vi "xiCMNG - Manager.vi"(6 "xiCam":refnum<k24>, 7 "States":T1, 8 "error in (no error)":errorcluster, 10 "SubPnl":refnum<vi>, 11 "xiControlPath":path) -> (0 "error out":errorcluster, 3 "StatusOut":T2)   [LabVIEW 2013]
doc: "xiControl Manger. Action Engine for xiControl panel."
uses:
  xiCMNG - States.ctl
  xiCMNG - Attributes.ctl
  C:/Projects/Cameras3.x/xiLib/xiLIB_64bit/xiLIB/xiCamLib/API/x64/xiApi.NETX64.dll
  xiLIB_64bit/xiLIB/xiCamLib/API/x64/xiApi.NETX64.dll
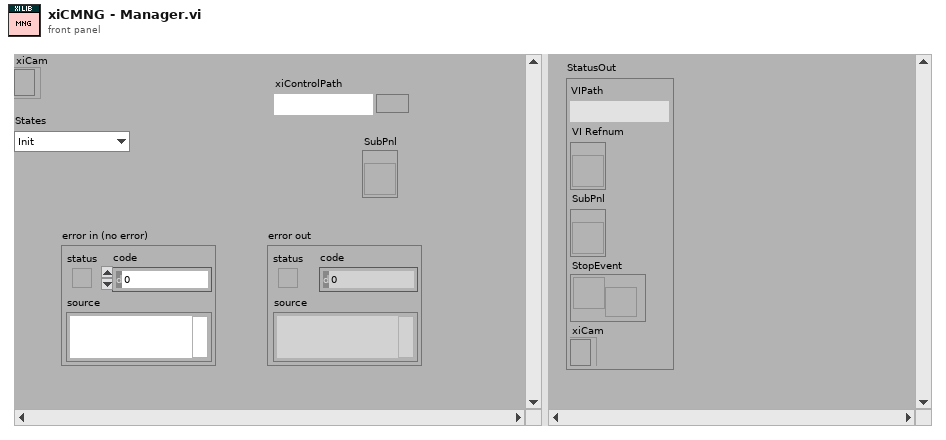
[diagram p1: front panel]
types:
  T1 = typedef "xiCMNG - States.ctl" = enum16{"Init", "Open", "Close", "Status"}
  T2 = typedef "xiCMNG - Attributes.ctl" = cluster{"VIPath":path, "VI Refnum":refnum<vi>, "SubPnl":refnum<vi>, "StopEvent":refnum<user-event>, "xiCam":refnum<k24>}
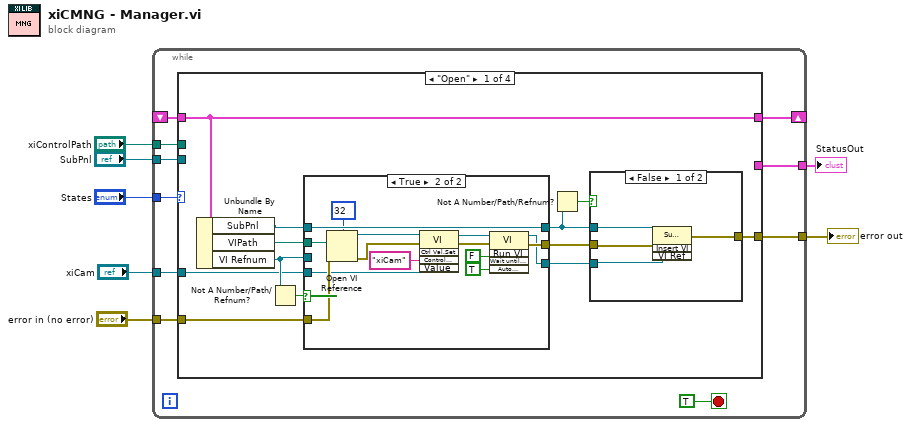
[diagram p0: block diagram]
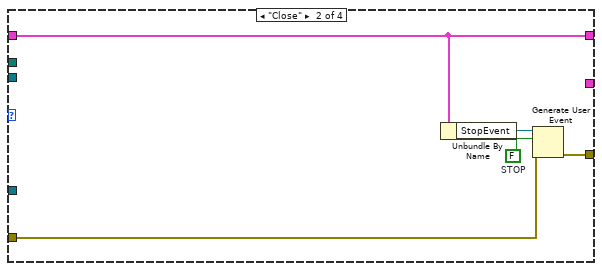
[diagram p4: hidden frame]
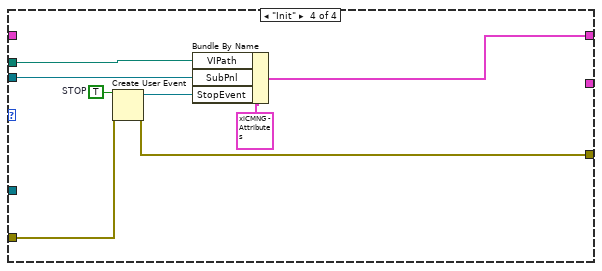
[diagram p6: hidden frame]
diagram:
  n1 = while {
    shift-right: [w16] -> _
    shift-left: _ -> [w10]
    tunnel: "States" -> [w15]
    tunnel: "error in (no error)" -> [w14]
    tunnel: [w13] -> w5
    tunnel: "SubPnl" -> [w12]
    tunnel: "xiControlPath" -> [w11]
    tunnel: [w9] -> w2
    tunnel: "xiCam" -> [w8]
    stop <- TRUE stop-if-true
    n2 = case shown="\"Open\"" w15 {
      tunnel: [w29 w56 w58 w63] -> w16
      tunnel: w14 -> [w26 w54 w57 w65]
      tunnel: [w19 w53 w57 w64] -> w13
      tunnel: w12 -> [_ _ _ w60]
      tunnel: w11 -> [_ _ _ w59]
      tunnel: w10 -> [w29 w56 w58 _]
      tunnel: [_ _ w58 _] -> w9
      tunnel: w8 -> [w18 _ _ _]
      frame "Open" {
        n3 = Unbundle By Name(w29) -> ("SubPnl"=w25:refnum<vi>, "VIPath"=w27:path, "VI Refnum"=w24:refnum<vi>)
        n4 = Not A Number/Path/Refnum?(number/path/refnum=w24) -> (NaN/Path/Refnum?=w28:bool)
        n5 = case shown="True" w28 {
          tunnel: w27 -> [_ w51]
          tunnel: w26 -> [w35 w50]
          tunnel: w25 -> [w36 w49]
          tunnel: [w36 w49] -> w22
          tunnel: [w37 w39] -> w20
          tunnel: w24 -> [w37 _]
          tunnel: [w35 w40] -> w21
          tunnel: w18 -> [_ w44]
          frame False {
          }
          frame True {
            n6 = Open VI Reference(vi path=w51, options=32, error in (no error)=w50) -> (vi reference=w47:refnum<vi>, error out=w46:errorcluster)  [unwired: 3 in]
            n7 = invoke class="VI" method="Ctrl Val.Set"(reference=w47, error in=w46, "Control Name"="xiCam", "Value"=w44) -> (reference out=w41:refnum<vi>, error out=w42:errorcluster)  [unwired: 1 in, 3 out]
            n8 = invoke class="VI" method="Run VI"(reference=w41, error in=w42, "Wait until done"=FALSE ("Wait Until Done"), "Auto Dispose Ref"=TRUE ("Auto Dispose Reference")) -> (reference out=w39:refnum<vi>, error out=w40:errorcluster)  [unwired: 1 in, 3 out]
          }
        }
        n9 = Not A Number/Path/Refnum?(number/path/refnum=w22) -> (NaN/Path/Refnum?=w23:bool)
        n10 = case shown="False" w23 {
          tunnel: w22 -> [w33 _]
          tunnel: w21 -> [w32 w34]
          tunnel: w20 -> [w31 _]
          tunnel: [w30 w34] -> w19
          frame False {
            n11 = invoke class="SubPnl" method="Insert VI"(reference=w33, error in=w32, "VI Ref"=w31) -> (error out=w30:errorcluster)  [unwired: 1 in, 3 out]
          }
          frame True {
          }
        }
      }
      frame "Close" {
        w52 = FALSE  # STOP
        n12 = Unbundle By Name(w56) -> ("StopEvent"=w55:refnum<user-event>)
        n13 = Generate User Event(user event=w55, event data cluster=w52, error in=w54) -> (error out=w53:errorcluster)  [unwired: 1 in, 1 out]
      }
      frame "Status" {
      }
      frame "Init" {
        w66 = TRUE  # STOP
        n14 = Create User Event(user event datatype=w66, error in=w65) -> (user event=w61:refnum<user-event>, error out=w64:errorcluster)
        n15 = Bundle By Name(cluster=T2 {"VIPath"=path "", "VI Refnum"=refnum, "SubPnl"=refnum, "StopEvent"=refnum, "xiCam"=refnum} ("Attributes"), "VIPath"=w59, "SubPnl"=w60, "StopEvent"=w61) -> (w63:T2)
      }
    }
  }
  "error out" <- w5
  "StatusOut" <- w2
